vi "Drawing Images.vi"() -> ()   [LabVIEW 2020]
uses:
  d1d740a6-f6ea-48db-ad8b-37ffab3f668f.vi
panel:
  in  "Zoom?":bool
  in  "Window Size":dbl
  in  "Image":T1(ring)
  out "Current Time":dbl
  out "XY Graph":cluster{dbl[], dbl[]}[](graph)
  in  "stop":bool
  in  "Period":dbl
  in  "Number of Terms":dbl
  in  "Draw Circle?":bool
  # "Drawing Settings"
  # "Zoom Options"
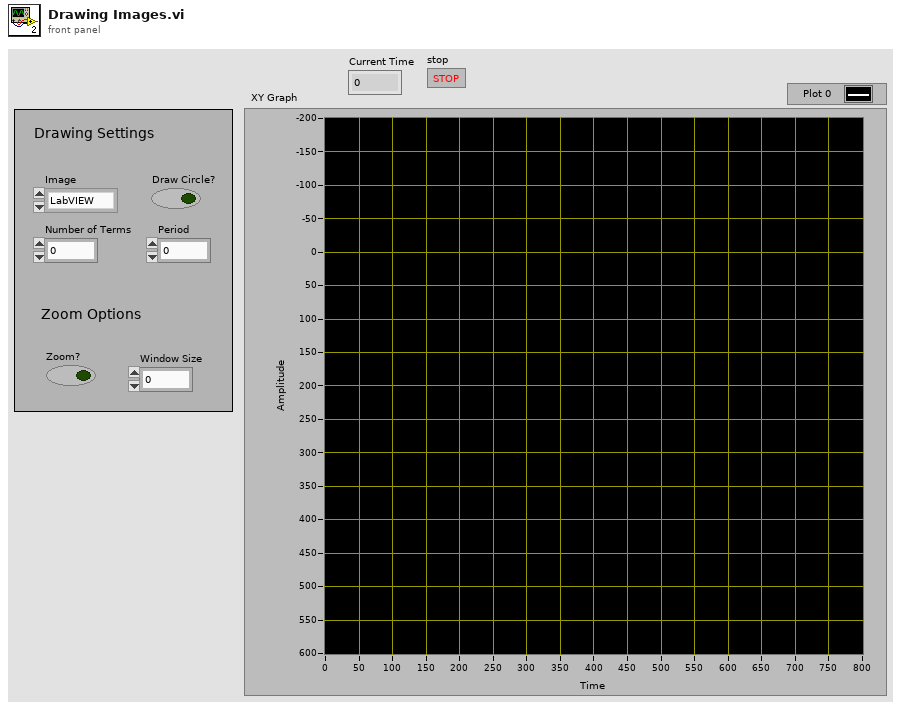
[diagram p1: front panel]
types:
  T1 = enum16{"LabVIEW", "Sphagett", "Treble Cleff", "FRC", "Cricket Bat", "Troll Face", "Rick Astley"}
  T2 = typedef "Component.ctl" = cluster{"Radius Formula":string, "Frequency":dbl, "Phase Offset":dbl}
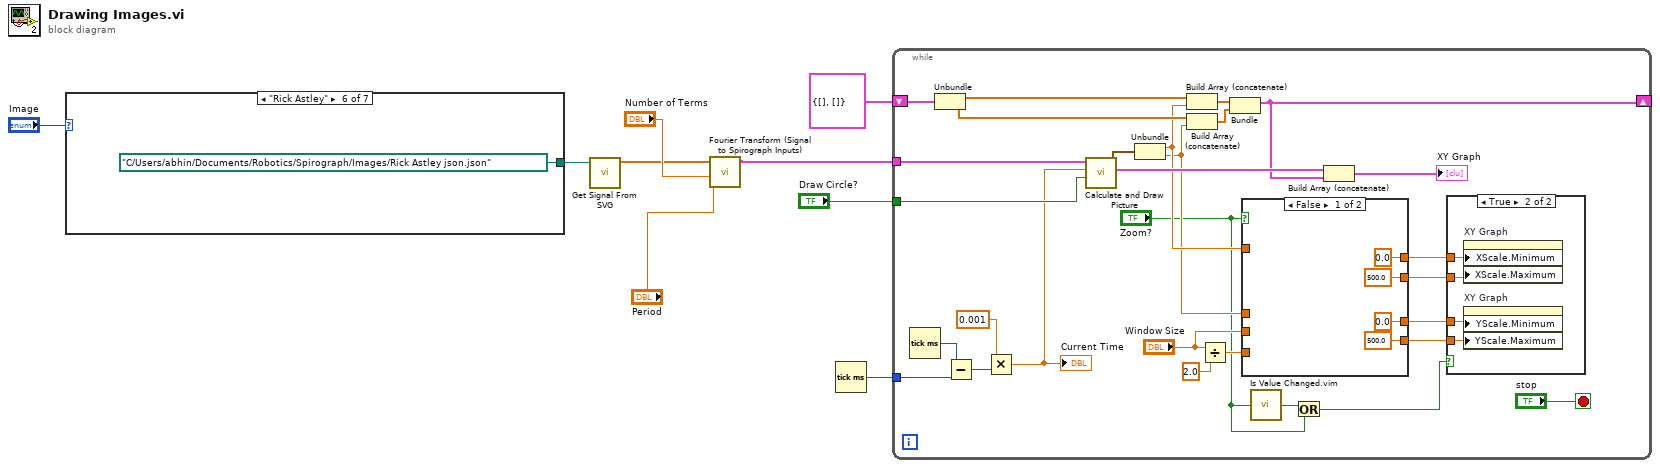
[diagram p0: block diagram]
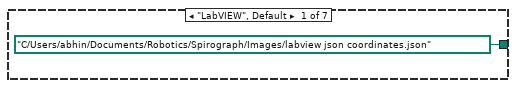
[diagram p2: hidden frame]
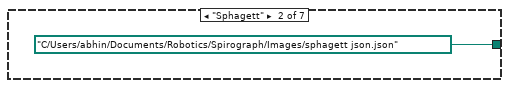
[diagram p3: hidden frame]
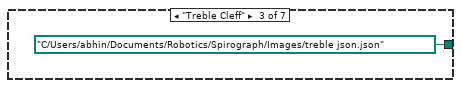
[diagram p4: hidden frame]
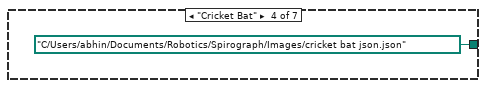
[diagram p5: hidden frame]
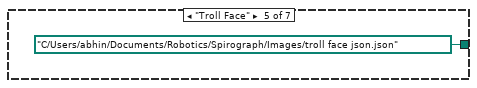
[diagram p6: hidden frame]
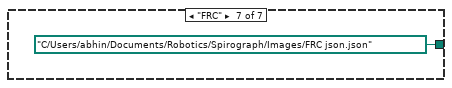
[diagram p7: hidden frame]
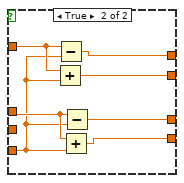
[diagram p9: hidden frame]
diagram:
  n1 = case shown="\"Rick Astley\"" "Image" {
    tunnel: [path "C:/Users/abhin/Documents/Robotics/Spirograph/Images/labview json coordinates.json" ("file path (use dialog)") path "C:/Users/abhin/Documents/Robotics/Spirograph/Images/sphagett json.json" ("file path (use dialog)") path "C:/Users/abhin/Documents/Robotics/Spirograph/Images/treble json.json" ("file path (use dialog)") path "C:/Users/abhin/Documents/Robotics/Spirograph/Images/cricket bat json.json" ("file path (use dialog)") path "C:/Users/abhin/Documents/Robotics/Spirograph/Images/troll face json.json" ("file path (use dialog)") path "C:/Users/abhin/Documents/Robotics/Spirograph/Images/Rick Astley json.json" ("file path (use dialog)") path "C:/Users/abhin/Documents/Robotics/Spirograph/Images/FRC json.json" ("file path (use dialog)")] -> w1
    frame "LabVIEW", Default {
    }
    frame "Sphagett" {
    }
    frame "Treble Cleff" {
    }
    frame "Cricket Bat" {
    }
    frame "Troll Face" {
    }
    frame "Rick Astley" {
    }
    frame "FRC" {
    }
  }
  n2 = call "Get Signal From SVG.vi"("file path (use dialog)"=w1) -> ("Signal"=w3:cdb[])  [unwired: 10 in]
  n3 = call "Fourier Transform (Signal to Spirograph Inputs).vi"("Number of Terms"="Number of Terms", "Period"="Period", "Signal"=w3) -> ("Inputs"=w7:T2[])  [unwired: 8 in]
  n4 = Tick Count (ms)() -> (millisecond timer value=w9:u32)
  n5 = while {
    tunnel: w7 -> [w42]
    tunnel: w9 -> [w45]
    tunnel: "Draw Circle?" -> [w43]
    shift-right: [w32] -> _
    shift-left: cluster{dbl[], dbl[]} {[], []} -> [w38]
    stop <- "stop" stop-if-true
    n6 = Tick Count (ms)() -> (millisecond timer value=w44:u32)
    n7 = Unbundle(w38) -> (w37:dbl[], w36:dbl[])
    n8 = Subtract(x=w44, y=w45) -> (x-y=w41:u32)
    n9 = Multiply(x=0.001, y=w41) -> (x*y=w31:dbl)
    "Current Time" <- w31
    n10 = call "Calculate and Draw Picture.vi"("Draw Circle?"=w43, "Time"=w31, "Inputs"=w42) -> ("Points"=w33:cluster{dbl[], dbl[]}[], "Endpoint"=w39:cluster{"x":dbl, "y":dbl})  [unwired: 7 in]
    n11 = Unbundle(w39) -> ("x"=w26:dbl, "y"=w25:dbl)
    n12 = Build Array (concatenate)(w37, w26) -> (w35:dbl[])
    n13 = Build Array (concatenate)(w36, w25) -> (w34:dbl[])
    n14 = Divide(x="Window Size", y=2.0) -> (x/y=w27:dbl)
    n15 = Bundle(w35, w34) -> (w32:cluster{dbl[], dbl[]})  [unwired: 1 in]
    n16 = case shown="False" "Zoom?" {
      tunnel: w27 -> [_ w58]
      tunnel: w26 -> [_ w60]
      tunnel: w25 -> [_ w59]
      tunnel: [0.0 w57] -> w24
      tunnel: [500.0 w56] -> w23
      tunnel: [0.0 w55] -> w22
      tunnel: [500.0 w54] -> w21
      tunnel: "Window Size" -> [_ _]
      frame False {
      }
      frame True {
        n17 = Add(x=w60, y=w58) -> (x+y=w54:dbl)
        n18 = Subtract(x=w60, y=w58) -> (x-y=w55:dbl)
        n19 = Add(x=w59, y=w58) -> (x+y=w56:dbl)
        n20 = Subtract(x=w59, y=w58) -> (x-y=w57:dbl)
      }
    }
    n21 = call "Is Value Changed.vim"("value"="Zoom?") -> ("changed or first call?"=w19:bool)
    n22 = Or(x=w19, y="Zoom?") -> (x .or. y?=w17:bool)
    n23 = Build Array (concatenate)(w33, w32) -> (→"XY Graph":cluster{dbl[], dbl[]}[])
    n24 = case shown="True" w17 {
      tunnel: w24 -> [_ w49]
      tunnel: w23 -> [_ w48]
      tunnel: w22 -> [_ w47]
      tunnel: w21 -> [_ w46]
      frame False {
      }
      frame True {
        n25 = property on="XY Graph" class="XYGraph (strict)"("XScale.Minimum"=w47, "XScale.Maximum"=w46) -> ()  [unwired: 2 in, 2 out]
        n26 = property on="XY Graph" class="XYGraph (strict)"("YScale.Minimum"=w49, "YScale.Maximum"=w48) -> ()  [unwired: 2 in, 2 out]
      }
    }
  }
